vi "Decompose VI.vi"   [LabVIEW 2023, in "Resource Manipulation.lvlib"]
uses:
  Resource Manipulation.lvlib
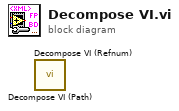
[diagram p0: block diagram]
diagram:
  n1 = call "Decompose VI (Path).vi"() -> ()  [unwired: 7 in, 5 out]
  n2 = call "Decompose VI (Refnum).vi"() -> ()  [unwired: 7 in, 5 out]
